vi "trigger-test2.vi"() -> ()   [LabVIEW 2020]
uses:
  <instrlib>/niDMM/nidmm.llb/niDMM Waveform Function.ctl
  <instrlib>/niDMM/nidmm.llb/niDMM Trigger.ctl
  Realization/PI650 VoltageAmp/TypeDefs/Channel gain.ctl
  Realization/PIPX40 Matrix/PIPX40 Matrix.lvclass
  Realization/PI650 VoltageAmp/PI650 VoltageAmp.lvclass
  Realization/PI650 VoltageAmp/TypeDefs/Channel DC offset.ctl
  Realization/NI Analog Output/NI Analog Output.lvclass
  Realization/NI DAQmx Base/TypeDefs/Channel Config.ctl
  Realization/NI Analog Output/TypeDefs/Timing Config.ctl
  Realization/NI Analog Output/TypeDefs/Trigger Config.ctl
  Realization/NI Analog Input/NI Analog Input.lvclass
  <vilib>/DAQmx/create/channels.llb/DAQmx Create Channel (CO-Pulse Generation-Frequency).vi
  <vilib>/DAQmx/configure/timing.llb/DAQmx Timing (Implicit).vi
  <instrlib>/niDMM/nidmm.llb/niDMM Fetch Waveform (waveform data).vi
  <vilib>/DAQmx/configure/timing.llb/DAQmx Timing (Sample Clock).vi
  <vilib>/DAQmx/configure/trigger.llb/DAQmx Start Trigger (Digital Edge).vi
  <vilib>/measure/NI_MABase.lvlib
  <vilib>/DAQmx/create/channels.llb/DAQmx Create Channel (AI-Voltage-Basic).vi
  <vilib>/DAQmx/read.llb/DAQmx Read (Analog 1D Wfm NChan NSamp).vi
  <vilib>/DAQmx/write.llb/DAQmx Write (Analog 1D DBL 1Chan NSamp).vi
  <vilib>/DAQmx/create/channels.llb/DAQmx Create Channel (AO-Voltage-Basic).vi
panel:
  in  "Channel gain":T1={"Channel (CH1)"=3, "Gain (x1)"=2} {"Channel (CH1)" items=["CH1"=1, "CH2"=2, "CH3"=3, "CH4"=4, "CH5"=5]; "Gain (x1)" items=["x1"=1, "x2"=2, "x5"=3, "x7"=4, "x10"=5, "x14"=6, "x20"=7]}
  out "Amp Info":variant
  out "Mx infos":variant[](array[variant])
  in  "analog input":tag="NI_AnaIn1/ai0:1"
  in  "Trigger Source":T2=enum."TTL 0"
  in  "Function":T3=1003 items=["Waveform_Voltage"=1003, "Waveform_Current"=1004]
  in  "Device Name":refnum<k15>="NI_DMM"
  out "Waveform Graph":dynamicdata(graph)
  in  "counter output":tag="NI_Timing/ctr0"
  out "error out":errorcluster
  in  "source terminal":tag="/NI_Timing/PFI0"
  in  "destination terminal":tag="/NI_AnaIn1/PXI_Trig0"
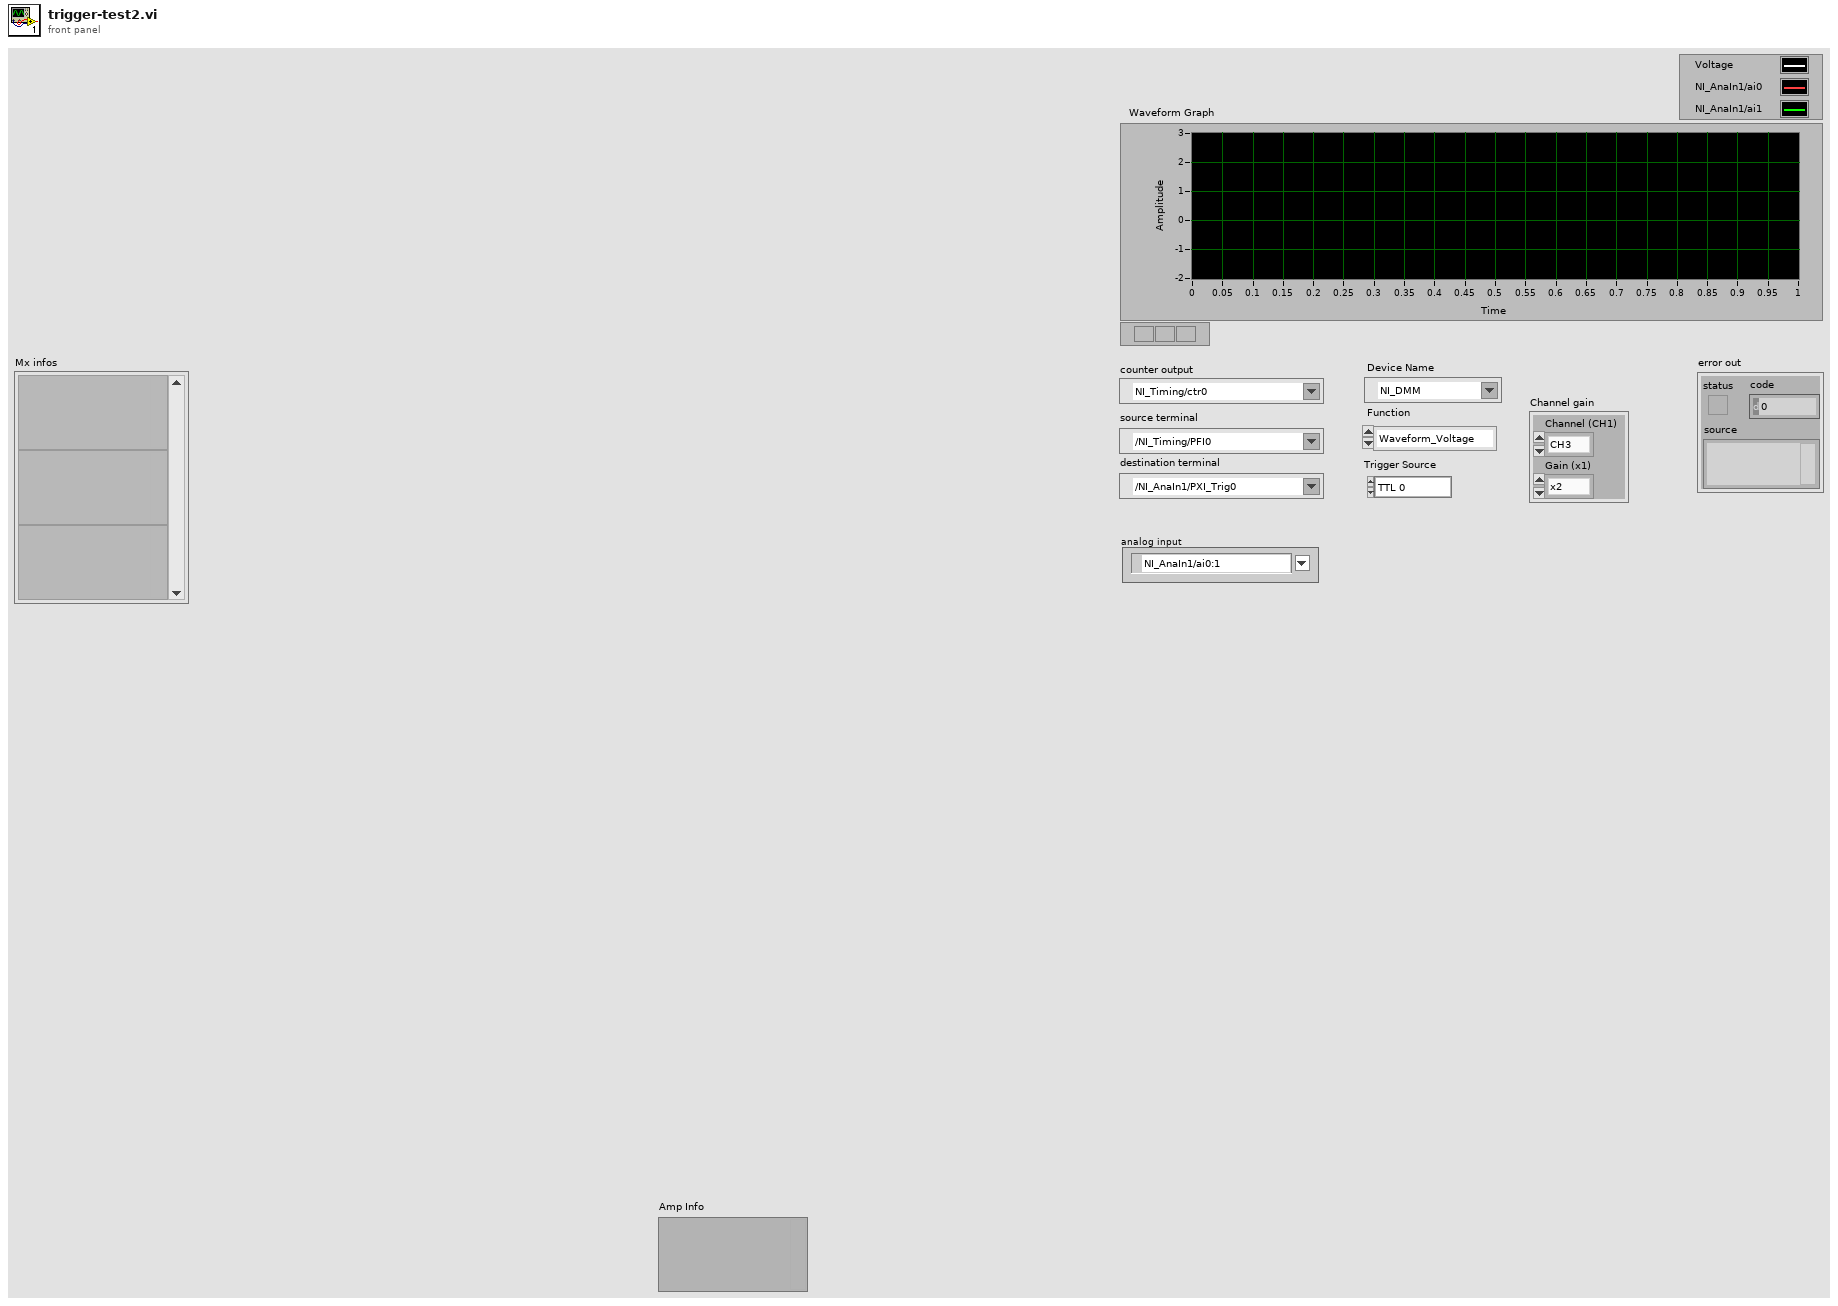
[diagram p1: front panel]
types:
  T1 = typedef "Channel gain.ctl" = cluster{"Channel (CH1)":u32, "Gain (x1)":u32}
  T2 = typedef "niDMM Trigger.ctl" = enum16{"Immediate", "External", "TTL 0", "TTL 1", "TTL 2", "TTL 3", "TTL 4", "TTL 5", "TTL 6", "Software", "TTL 7", "PXI Star", "LBR Trig 1", "Aux Trig 1"}
  T3 = typedef "niDMM Waveform Function.ctl" = i32
  T4 = typedef "Channel DC offset.ctl" = cluster{"Channel (CH1)":u32, "Offset (128)":u32}
  T5 = enum16{"Sine Wave", "Triangle Wave", "Square Wave", "Sawtooth Wave"}
  T6 = map{string, refnum<class "PIPX40 Matrix.lvclass">}
  T7 = cluster{"samples per channel":dbl, "samples per channel":dbl}
  T8 = typedef "Trigger Config.ctl" = cluster{"trigger type":string, "source":string, "slope":i32, "analog level":dbl, "analog hysteresis":dbl}
  T9 = typedef "Channel Config.ctl" = cluster{"channels":string, "maximum value":dbl, "minimum value":dbl, "output terminal configuration":i32, "units":i32}
  T10 = typedef "Timing Config.ctl" = cluster{"sample mode":i32, "samples per channel":i32, "rate":dbl, "source":string, "active edge":i32}
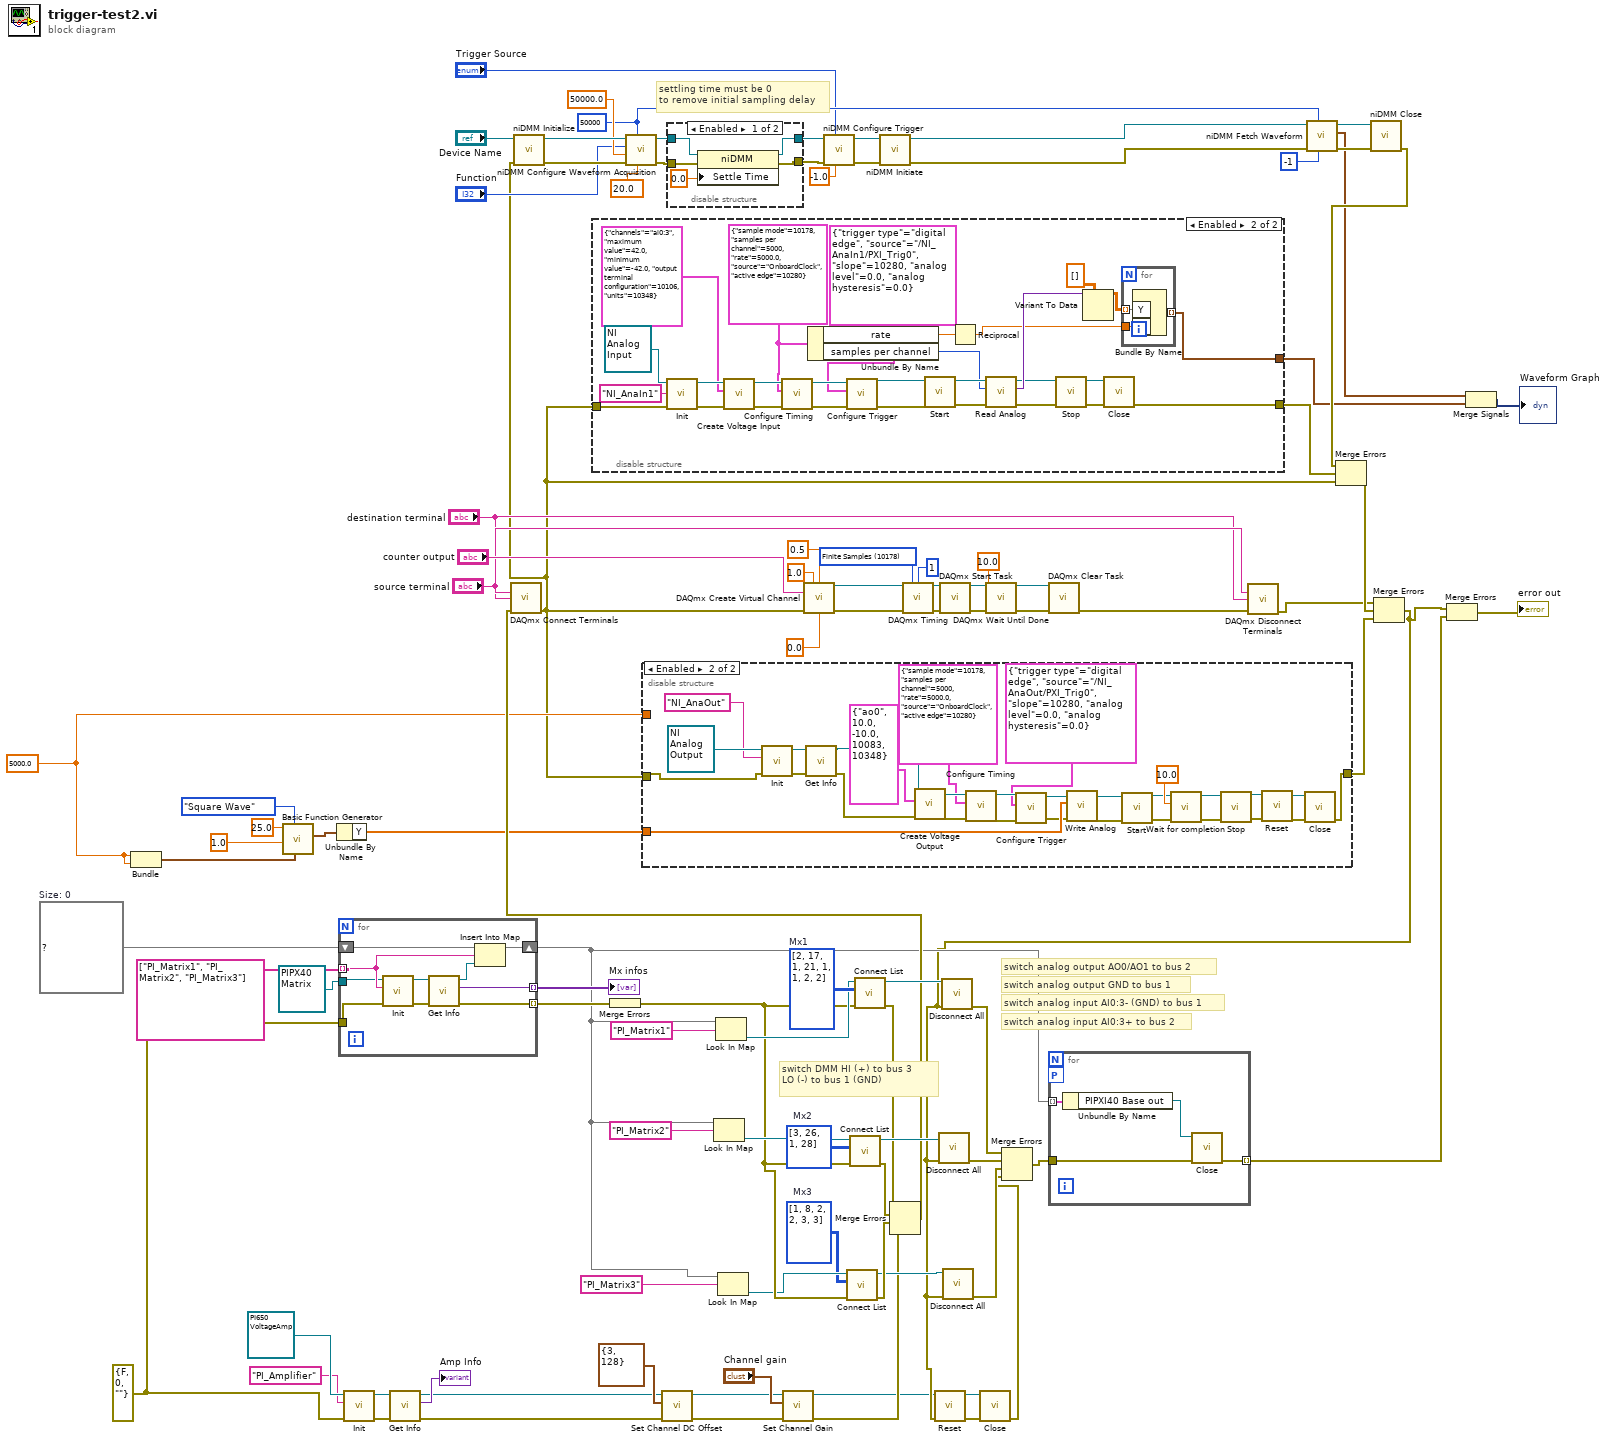
[diagram p0: block diagram]
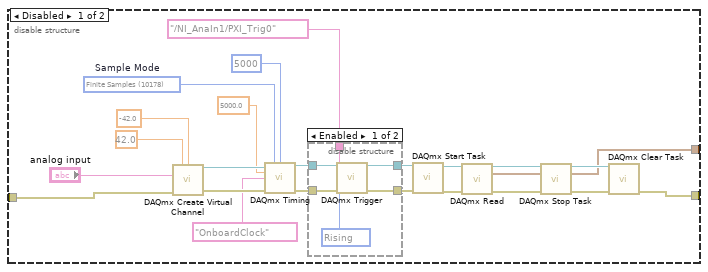
[diagram p3: hidden frame]
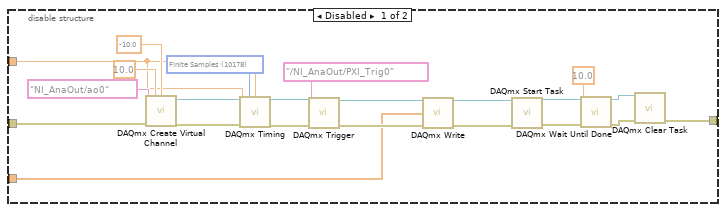
[diagram p5: hidden frame]
diagram:
  w22 = errorcluster {"status"=FALSE, "code"=0, "source"=""} ("error in (no error)")
  w33 = i32[][] [[1, 8], [2, 2], [3, 3]]  # Mx3
  w48 = T6 {}  # Size: 0
  w57 = i32[][] [[3, 26], [1, 28]]  # Mx2
  w59 = i32[][] [[2, 17], [1, 21], [1, 1], [2, 2]]  # Mx1
  w39 = 5000.0 ("samples per channel")
  w71 = 10178 items=["Finite Samples"=10178, "Continuous Samples"=10123, "Hardware Timed Single Point"=12522] ("sample mode")
  w92 = 50000 ("Number of samples")
  # "settling time must be 0\nto remove initial sampling delay"
  # "switch analog input AI0:3+ to bus 2"
  # "switch analog input AI0:3- (GND) to bus 1"
  # "switch analog output GND to bus 1"
  # "switch analog output AO0/AO1 to bus 2"
  # "switch DMM HI (+) to bus 3 \nLO (-) to bus 1 (GND)"
  n1 = Bundle("samples per channel"=w39, "samples per channel"=w39) -> (w38:T7)  [unwired: 1 in]
  n2 = call <vilib>:"Basic Function Generator.vi"("sampling info"=w38, "signal type"=T5."Square Wave", "amplitude"=1.0, "frequency"=25.0) -> ("signal out"=w11:waveform(dbl))  [unwired: 5 in, 2 out]
  n3 = Unbundle By Name(w11) -> ("Y"=w10:dbl[])
  n4 = for {
    tunnel: string[] ["PI_Matrix1", "PI_Matrix2", "PI_Matrix3"] -> [w107] mode=indexing
    tunnel: [w110] -> w62 mode=indexing
    tunnel: [w109] -> w61 mode=indexing
    shift-right: [w108] -> w36
    shift-left: w48 -> [w105]
    tunnel: refnum<class "PIPX40 Matrix.lvclass"> refnum ("PIPXI40 Matrix in") -> [w103]
    tunnel: w22 -> [w102]
    n5 = call-dynamic "Init.vi"("error in (no error)"=w102, "Params"=w107, "PIPXI40 Base in"=w103) -> ("error out"=w111:errorcluster, "PIPXI40 Base out"=w106:refnum<class "PIPX40 Matrix.lvclass">)  [unwired: 7 in]
    n6 = call-dynamic "Get Info.vi"("error in (no error)"=w111, "PIPXI40 Base in"=w106) -> ("error out"=w110:errorcluster, "Info"=w109:variant, "PIPXI40 Base out"=w104:refnum<class "PIPX40 Matrix.lvclass">)  [unwired: 7 in]
    n7 = Insert Into Map(map in=w105, key=w107, value=w104) -> (map out=w108:T6)  [unwired: 2 out]
  }
  "Mx infos" <- w61
  n8 = call-dynamic "Init.vi"("error in (no error)"=w22, "Params"="PI_Amplifier" ("String"), "PI650 VoltageAmp in"=refnum<class "PI650 VoltageAmp.lvclass"> refnum) -> ("error out"=w27:errorcluster, "PI650 VoltageAmp out"=w28:refnum<class "PI650 VoltageAmp.lvclass">)  [unwired: 7 in]
  n9 = call-dynamic "Get Info.vi"("error in (no error)"=w27, "PI650 VoltageAmp in"=w28) -> ("error out"=w21:errorcluster, "Info"=→"Amp Info":variant, "PI650 VoltageAmp out"=w20:refnum<class "PI650 VoltageAmp.lvclass">)  [unwired: 7 in]
  n10 = Merge Errors(w62) -> (w35:errorcluster)
  n11 = call-dynamic "Set Channel DC Offset.vi"("error in (no error)"=w21, "Params"=T4 {"Channel (CH1)"=3, "Offset (128)"=128}, "PI650 VoltageAmp in"=w20) -> ("error out"=w18:errorcluster, "PI650 VoltageAmp out"=w19:refnum<class "PI650 VoltageAmp.lvclass">)  [unwired: 7 in]
  n12 = Look In Map(map=w36, key="PI_Matrix2" ("String")) -> (value=w50:refnum<class "PIPX40 Matrix.lvclass">)  [unwired: 1 in, 1 out]
  n13 = Look In Map(map=w36, key="PI_Matrix1" ("String")) -> (value=w51:refnum<class "PIPX40 Matrix.lvclass">)  [unwired: 1 in, 1 out]
  n14 = Look In Map(map=w36, key="PI_Matrix3" ("String")) -> (value=w34:refnum<class "PIPX40 Matrix.lvclass">)  [unwired: 1 in, 1 out]
  n15 = call-dynamic "Set Channel Gain.vi"("error in (no error)"=w18, "Params"="Channel gain", "PI650 VoltageAmp in"=w19) -> ("error out"=w17:errorcluster, "PI650 VoltageAmp out"=w13:refnum<class "PI650 VoltageAmp.lvclass">)  [unwired: 7 in]
  n16 = call-dynamic "Connect List.vi"("error in (no error)"=w35, "Params"=w33, "PIPXI40 Matrix in"=w34) -> ("error out"=w32:errorcluster, "PIPXI40 Matrix out"=w31:refnum<class "PIPX40 Matrix.lvclass">)  [unwired: 7 in]
  n17 = call-dynamic "Connect List.vi"("error in (no error)"=w35, "Params"=w57, "PIPXI40 Matrix in"=w50) -> ("error out"=w46:errorcluster, "PIPXI40 Matrix out"=w55:refnum<class "PIPX40 Matrix.lvclass">)  [unwired: 7 in]
  n18 = call-dynamic "Connect List.vi"("error in (no error)"=w35, "Params"=w59, "PIPXI40 Matrix in"=w51) -> ("error out"=w47:errorcluster, "PIPXI40 Matrix out"=w56:refnum<class "PIPX40 Matrix.lvclass">)  [unwired: 7 in]
  n19 = Merge Errors(w47, w46, w32, w17) -> (w45:errorcluster)
  n20 = call <vilib>:"DAQmx Connect Terminals.vi"("source terminal"="source terminal", "destination terminal"="destination terminal", "error in"=w45) -> ("error out"=w2:errorcluster)  [unwired: 12 in]
  n21 = call <instrlib>:"niDMM Initialize.vi"("error in (no error)"=w2, "Instrument Descriptor"="Device Name") -> ("error out"=w97:errorcluster, "instrument handle out"=w98:refnum<k15>)  [unwired: 8 in]
  n22 = disable-structure shown="Enabled" {
    disable-tunnel: [w117 w149] -> w65
    disable-tunnel: [w116 w143] -> w1
    disable-tunnel: w2 -> [w112 w163]
    frame Disabled {
      w132 = 10178 items=["Finite Samples"=10178, "Continuous Samples"=10123, "Hardware Timed Single Point"=12522]  # Sample Mode
      n23 = call-poly <vilib>:"DAQmx Create Virtual Channel.vi"("maximum value"=42.0 ("Max Voltage"), "minimum value"=-42.0 ("Min Voltage"), "physical channels"="analog input", "error in"=w112) -> ("task out"=w130:refnum<k21>, "error out"=w131:errorcluster)  [unwired: 10 in]
      n24 = call-poly <vilib>:"DAQmx Timing.vi"("task/channels in"=w130, "sample mode"=w132, "samples per channel"=5000 ("Number of Samples"), "rate"=5000.0 ("Sample Rate"), "source"=tag "OnboardClock" ("Sample Clock Source"), "error in"=w131) -> ("task out"=w134:refnum<k21>, "error out"=w133:errorcluster)  [unwired: 8 in]
      n25 = disable-structure shown="Enabled" {
        disable-tunnel: w134 -> [w140 w142]
        disable-tunnel: w133 -> [w139 w141]
        disable-tunnel: [w138 w142] -> w114
        disable-tunnel: [w137 w141] -> w120
        disable-tunnel: tag "/NI_AnaIn1/PXI_Trig0" ("source") -> [w136 _]
        frame Enabled {
          w135 = 10280 items=["Rising"=10280, "Falling"=10171] ("edge")
          n26 = call-poly <vilib>:"DAQmx Trigger.vi"("task/channels in"=w140, "source"=w136, "edge"=w135, "error in"=w139) -> ("task out"=w138:refnum<k21>, "error out"=w137:errorcluster)  [unwired: 10 in]
        }
        frame Disabled {
        }
      }
      n27 = call <vilib>:"DAQmx Start Task.vi"("task/channels in"=w114, "error in"=w120) -> ("task out"=w113:refnum<k21>, "error out"=w129:errorcluster)  [unwired: 12 in]
      n28 = call-poly <vilib>:"DAQmx Read.vi"("task/channels in"=w113, "error in"=w129) -> ("task out"=w122:refnum<k21>, "data"=w116:waveform(dbl)[], "error out"=w121:errorcluster)  [unwired: 11 in]
      n29 = call <vilib>:"DAQmx Stop Task.vi"("task/channels in"=w122, "error in"=w121) -> ("task out"=w124:refnum<k21>, "error out"=w123:errorcluster)  [unwired: 12 in]
      n30 = call <vilib>:"DAQmx Clear Task.vi"("task in"=w124, "error in"=w123) -> ("error out"=w117:errorcluster)  [unwired: 13 in]
    }
    frame Enabled {
      w147 = T10 {"sample mode"=10178, "samples per channel"=5000, "rate"=5000.0, "source"="OnboardClock", "active edge"=10280}
      n31 = call-dynamic "Init.vi"("error in (no error)"=w163, "Params"="NI_AnaIn1" ("String"), "DAQmx Base in"=refnum<class "NI Analog Input.lvclass"> refnum ("NI Analog Input in")) -> ("error out"=w169:errorcluster, "DAQmx Base out"=w168:refnum<class "NI Analog Input.lvclass">)  [unwired: 7 in]
      n32 = call-dynamic "Create Voltage Input.vi"("error in (no error)"=w169, "Params"=T9 {"channels"="ai0:3", "maximum value"=42.0, "minimum value"=-42.0, "output terminal configuration"=10106, "units"=10348} ("Channel Config"), "NI Analog Input in"=w168) -> ("error out"=w170:errorcluster, "NI Analog Input out"=w167:refnum<class "NI Analog Input.lvclass">)  [unwired: 7 in]
      n33 = call-dynamic "Configure Timing.vi"("error in (no error)"=w170, "Params"=w147, "NI DAQmx Base in"=w167) -> ("error out"=w165:errorcluster, "NI DAQmx Base out"=w166:refnum<class "NI Analog Input.lvclass">)  [unwired: 7 in]
      n34 = Unbundle By Name(w147) -> ("rate"=w145:dbl, "samples per channel"=w146:i32)
      n35 = call-dynamic "Configure Trigger.vi"("error in (no error)"=w165, "Params"=T8 {"trigger type"="digital edge", "source"="/NI_AnaIn1/PXI_Trig0", "slope"=10280, "analog level"=0.0, "analog hysteresis"=0.0}, "NI DAQmx Base in"=w166) -> ("error out"=w158:errorcluster, "NI DAQmx Base out"=w157:refnum<class "NI Analog Input.lvclass">)  [unwired: 7 in]
      n36 = call-dynamic "Start.vi"("error in (no error)"=w158, "NI DAQmx Base in"=w157) -> ("error out"=w159:errorcluster, "NI DAQmx Base out"=w156:refnum<class "NI Analog Input.lvclass">)  [unwired: 8 in]
      n37 = Reciprocal(x=w145) -> (1/x=w144:dbl)
      n38 = call-dynamic "Read Analog.vi"("error in (no error)"=w159, "Params"=w146, "NI Analog Input in"=w156) -> ("error out"=w151:errorcluster, "Data"=w154:variant, "NI Analog Input out"=w152:refnum<class "NI Analog Input.lvclass">)  [unwired: 6 in]
      n39 = call-dynamic "Stop.vi"("error in (no error)"=w151, "NI DAQmx Base in"=w152) -> ("error out"=w150:errorcluster, "NI DAQmx Base out"=w153:refnum<class "NI Analog Input.lvclass">)  [unwired: 8 in]
      n40 = Variant To Data(type=dbl[][] [], Variant=w154) -> (data=w148:dbl[][])  [unwired: 1 in, 1 out]
      n41 = call-dynamic "Close.vi"("error in (no error)"=w150, "DAQmx Base in"=w153) -> ("error out"=w149:errorcluster)  [unwired: 8 in, 1 out]
      n42 = for {
        tunnel: w148 -> [w173] mode=indexing
        tunnel: [w172] -> w143 mode=indexing
        tunnel: w144 -> [w171]
        n43 = Bundle By Name("Y"=w173, "dt"=w171) -> (w172:waveform(dbl))  [unwired: 1 in]
      }
    }
  }
  n44 = call <instrlib>:"niDMM Configure Waveform Acquisition.vi"("Range"=20.0, "Waveform Points"=w92, "error in (no error)"=w97, "Rate"=50000.0 ("Sample Rate"), "Function"="Function", "instrument handle"=w98) -> ("error out"=w6:errorcluster, "instrument handle out"=w5:refnum<k15>)  [unwired: 4 in]
  n45 = disable-structure shown="Enabled" {
    disable-tunnel: w2 -> [w194 w220]
    disable-tunnel: [w176 w202] -> w64
    disable-tunnel: w39 -> [w175 _]
    disable-tunnel: w10 -> [w174 w214]
    frame Disabled {
      w189 = 10178 items=["Finite Samples"=10178, "Continuous Samples"=10123, "Hardware Timed Single Point"=12522] ("sample mode")
      n46 = call-poly <vilib>:"DAQmx Create Virtual Channel.vi"("maximum value"=10.0, "minimum value"=-10.0, "physical channels"=tag "NI_AnaOut/ao0", "error in"=w194) -> ("task out"=w190:refnum<k21>, "error out"=w191:errorcluster)  [unwired: 10 in]
      n47 = call-poly <vilib>:"DAQmx Timing.vi"("task/channels in"=w190, "sample mode"=w189, "samples per channel"=w175, "rate"=w175, "error in"=w191) -> ("task out"=w185:refnum<k21>, "error out"=w186:errorcluster)  [unwired: 9 in]
      n48 = call-poly <vilib>:"DAQmx Trigger.vi"("task/channels in"=w185, "source"=tag "/NI_AnaOut/PXI_Trig0", "error in"=w186) -> ("task out"=w183:refnum<k21>, "error out"=w182:errorcluster)  [unwired: 11 in]
      n49 = call-poly <vilib>:"DAQmx Write.vi"("task/channels in"=w183, "data"=w174, "error in"=w182) -> ("task out"=w187:refnum<k21>, "error out"=w188:errorcluster)  [unwired: 10 in, 1 out]
      n50 = call <vilib>:"DAQmx Start Task.vi"("task/channels in"=w187, "error in"=w188) -> ("task out"=w179:refnum<k21>, "error out"=w180:errorcluster)  [unwired: 12 in]
      n51 = call <vilib>:"DAQmx Wait Until Done.vi"("task/channels in"=w179, "timeout (sec)"=10.0, "error in"=w180) -> ("task out"=w178:refnum<k21>, "error out"=w177:errorcluster)  [unwired: 11 in]
      n52 = call <vilib>:"DAQmx Clear Task.vi"("task in"=w178, "error in"=w177) -> ("error out"=w176:errorcluster)  [unwired: 13 in]
    }
    frame Enabled {
      n53 = call-dynamic "Init.vi"("error in (no error)"=w220, "Params"="NI_AnaOut" ("String"), "DAQmx Base in"=refnum<class "NI Analog Output.lvclass"> refnum ("NI DAQmx.lvlib:NI Analog Output.lvclass")) -> ("error out"=w222:errorcluster, "DAQmx Base out"=w223:refnum<class "NI Analog Output.lvclass">)  [unwired: 7 in]
      n54 = call-dynamic "Get Info.vi"("error in (no error)"=w222, "DAQmx Base in"=w223) -> ("error out"=w196:errorcluster, "DAQmx Base out"=w218:refnum<class "NI Analog Output.lvclass">)  [unwired: 7 in, 1 out]
      n55 = call-dynamic "Create Voltage Output.vi"("error in (no error)"=w196, "Params"=T9 {"channels"="ao0", "maximum value"=10.0, "minimum value"=-10.0, "output terminal configuration"=10083, "units"=10348} ("Channel Config"), "NI Analog Output in"=w218) -> ("error out"=w217:errorcluster, "NI Analog Output out"=w216:refnum<class "NI Analog Output.lvclass">)  [unwired: 7 in]
      n56 = call-dynamic "Configure Timing.vi"("error in (no error)"=w217, "Params"=T10 {"sample mode"=10178, "samples per channel"=5000, "rate"=5000.0, "source"="OnboardClock", "active edge"=10280}, "NI DAQmx Base in"=w216) -> ("error out"=w201:errorcluster, "NI DAQmx Base out"=w200:refnum<class "NI Analog Output.lvclass">)  [unwired: 7 in]
      n57 = call-dynamic "Configure Trigger.vi"("error in (no error)"=w201, "Params"=T8 {"trigger type"="digital edge", "source"="/NI_AnaOut/PXI_Trig0", "slope"=10280, "analog level"=0.0, "analog hysteresis"=0.0}, "NI DAQmx Base in"=w200) -> ("error out"=w198:errorcluster, "NI DAQmx Base out"=w199:refnum<class "NI Analog Output.lvclass">)  [unwired: 7 in]
      n58 = call-dynamic "Write Analog.vi"("error in (no error)"=w198, "Params"=w214, "NI Analog Output in"=w199) -> ("error out"=w213:errorcluster, "NI Analog Output out"=w212:refnum<class "NI Analog Output.lvclass">)  [unwired: 7 in]
      n59 = call-dynamic "Start.vi"("error in (no error)"=w213, "NI DAQmx Base in"=w212) -> ("error out"=w206:errorcluster, "NI DAQmx Base out"=w205:refnum<class "NI Analog Output.lvclass">)  [unwired: 8 in]
      n60 = call-dynamic "Wait for completion.vi"("error in (no error)"=w206, "Params"=10.0, "NI DAQmx Base in"=w205) -> ("error out"=w208:errorcluster, "NI DAQmx Base out"=w209:refnum<class "NI Analog Output.lvclass">)  [unwired: 7 in]
      n61 = call-dynamic "Stop.vi"("error in (no error)"=w208, "NI DAQmx Base in"=w209) -> ("error out"=w211:errorcluster, "NI DAQmx Base out"=w210:refnum<class "NI Analog Output.lvclass">)  [unwired: 8 in]
      n62 = call-dynamic "Reset.vi"("error in (no error)"=w211, "DAQmx Base in"=w210) -> ("error out"=w204:errorcluster, "DAQmx Base out"=w203:refnum<class "NI Analog Output.lvclass">)  [unwired: 8 in]
      n63 = call-dynamic "Close.vi"("error in (no error)"=w204, "DAQmx Base in"=w203) -> ("error out"=w202:errorcluster)  [unwired: 8 in, 1 out]
    }
  }
  n64 = disable-structure shown="Enabled" {
    disable-tunnel: w6 -> [w229 w230]
    disable-tunnel: w5 -> [w228 w231]
    disable-tunnel: [w227 w231] -> w4
    disable-tunnel: [w226 w230] -> w3
    frame Enabled {
      n65 = property class="niDMM"(reference=w228, error in=w229, "Settle Time"=0.0 ("Configuration:Advanced:Settle Time")) -> (reference out=w227:refnum<k15>, error out=w226:errorcluster)
    }
    frame Disabled {
    }
  }
  n66 = call-poly <vilib>:"DAQmx Create Virtual Channel.vi"("frequency"=1.0, "duty cycle"=0.5, "counter"="counter output", "error in"=w2, "initial delay"=0.0) -> ("task out"=w69:refnum<k21>, "error out"=w70:errorcluster)  [unwired: 9 in]
  n67 = call <instrlib>:"niDMM Configure Trigger.vi"("Trigger Delay (sec)"=-1.0, "Trigger Source"="Trigger Source", "error in (no error)"=w3, "instrument handle"=w4) -> ("error out"=w89:errorcluster, "instrument handle out"=w90:refnum<k15>)  [unwired: 6 in]
  n68 = call <instrlib>:"niDMM Initiate.vi"("error in (no error)"=w89, "instrument handle"=w90) -> ("error out"=w87:errorcluster, "instrument handle out"=w7:refnum<k15>)  [unwired: 8 in]
  n69 = call-poly <vilib>:"DAQmx Timing.vi"("task/channels in"=w69, "sample mode"=w71, "samples per channel"=1, "error in"=w70) -> ("task out"=w79:refnum<k21>, "error out"=w80:errorcluster)  [unwired: 10 in]
  n70 = call <vilib>:"DAQmx Start Task.vi"("task/channels in"=w79, "error in"=w80) -> ("task out"=w77:refnum<k21>, "error out"=w78:errorcluster)  [unwired: 12 in]
  n71 = call <vilib>:"DAQmx Wait Until Done.vi"("task/channels in"=w77, "timeout (sec)"=10.0, "error in"=w78) -> ("task out"=w8:refnum<k21>, "error out"=w81:errorcluster)  [unwired: 11 in]
  n72 = call <vilib>:"DAQmx Clear Task.vi"("task in"=w8, "error in"=w81) -> ("error out"=w82:errorcluster)  [unwired: 13 in]
  n73 = call <vilib>:"DAQmx Disconnect Terminals.vi"("source terminal"="source terminal", "destination terminal"="destination terminal", "error in"=w82) -> ("error out"=w83:errorcluster)  [unwired: 12 in]
  n74 = call-poly <instrlib>:"niDMM Fetch Waveform.vi"("Maximum Time (msec)"=-1, "Number To Fetch"=w92, "error in (no error)"=w87, "instrument handle"=w7) -> ("error out"=w88:errorcluster, "Waveform Data"=w84:waveform(dbl), "instrument handle out"=w91:refnum<k15>)  [unwired: 4 in, 1 out]
  n75 = call <instrlib>:"niDMM Close.vi"("error in (no error)"=w88, "instrument handle"=w91) -> ("error out"=w85:errorcluster)  [unwired: 9 in]
  n76 = Merge Errors(w85, w65, w2) -> (w100:errorcluster)
  n77 = Merge Errors(w83, w100, w64) -> (w14:errorcluster)
  n78 = call-dynamic "Reset.vi"("error in (no error)"=w14, "PI650 VoltageAmp in"=w13) -> ("error out"=w15:errorcluster, "PI650 VoltageAmp out"=w16:refnum<class "PI650 VoltageAmp.lvclass">)  [unwired: 8 in]
  n79 = call-dynamic "Disconnect All.vi"("error in (no error)"=w14, "PIPXI40 Matrix in"=w55) -> ("error out"=w54:errorcluster)  [unwired: 8 in, 1 out]
  n80 = call-dynamic "Disconnect All.vi"("error in (no error)"=w14, "PIPXI40 Matrix in"=w56) -> ("error out"=w53:errorcluster)  [unwired: 8 in, 1 out]
  n81 = call-dynamic "Disconnect All.vi"("error in (no error)"=w14, "PIPXI40 Matrix in"=w31) -> ("error out"=w30:errorcluster)  [unwired: 8 in, 1 out]
  n82 = call-dynamic "Close.vi"("error in (no error)"=w15, "PI650 VoltageAmp in"=w16) -> ("error out"=w12:errorcluster)  [unwired: 8 in, 1 out]
  n83 = Merge Errors(w53, w54, w30, w12) -> (w52:errorcluster)
  n84 = for {
    tunnel: w52 -> [w234]
    tunnel: [w235] -> w44 mode=indexing
    workers-P: _ -> [_]
    tunnel: w36 -> [w233] mode=indexing
    n85 = Unbundle By Name(w233) -> ("PIPXI40 Base out"=w232:refnum<class "PIPX40 Matrix.lvclass">)
    n86 = call-dynamic "Close.vi"("error in (no error)"=w234, "PIPXI40 Base in"=w232) -> ("error out"=w235:errorcluster)  [unwired: 8 in, 1 out]
  }
  n87 = Merge Errors(w14, w44) -> (→"error out":errorcluster)
  n88 = Merge Signals(w84, w1) -> (→"Waveform Graph":dynamicdata)
